vi "Measure all pixels on cell and save data.vi"(0 "Cell details cluster in":T1={"Measure?"=TRUE, "Area (cm^2)"=0.0, "Cell Label"="", "Cell Description"="", "Cell Position"=0, "Time in rig (s)"=0.0, "Time to next scan (s)"=0.0, "Scan number"=0.0, "When did you stick it in?"=0.0, "Time between scans (s)"=0.0, "Time of the last scan (s)"=0.0, "Scan settings in queue"=0, "Sample Holder"=0.0} {"Scan settings in queue" items=["Regular", "Inverted"]; "Time of the last scan (s)" format="%<%H:%M:%S>t"; "When did you stick it in?" format="%<%H:%M:%S>t"; "Time to next scan (s)" format="%<%H:%M:%S>t"; "Time in rig (s)" format="%<%H:%M:%S>t"}, 1 "Username":string, 5 "Cell Description":string, 6 "XYGraph Refnum":refnum<vi>, 7 "Cell position":dbl, 8 "Tbl Refnum":refnum<vi>, 9 "Sample Holder":dbl, 11 "Scan settings in queue":dbl, 12 "JV curve scan settings":T2(array[cluster])=[{"Light Intensity (Suns)"=1.0, "Stabilization Time (s)"=2.0, "Maximum Voltage (V)"=0.0, "Minimum Voltage (V)"=-1.4, "Range Options"=0, "Scan Direction\nDU (T), UD (F)"=FALSE, "Step Size (V)"=0.01, "Source Delay (s)"=0.001}, {"Light Intensity (Suns)"=1.0, "Stabilization Time (s)"=5.0, "Maximum Voltage (V)"=2.0, "Minimum Voltage (V)"=0.0, "Range Options"=0, "Scan Direction\nDU (T), UD (F)"=TRUE, "Step Size (V)"=0.04, "Source Delay (s)"=0.001}] {"Range Options" items=["Auto Range", "Semi-Auto Range", "100 uA", "1 mA", "10 mA", "100 mA", "1A"]}, 13 "Time Zero":timestamp) -> (4 "Cell details cluster out":T1={"Measure?"=TRUE, "Area (cm^2)"=0.0, "Cell Label"="", "Cell Description"="", "Cell Position"=0, "Time in rig (s)"=0.0, "Time to next scan (s)"=0.0, "Scan number"=0.0, "When did you stick it in?"=0.0, "Time between scans (s)"=0.0, "Time of the last scan (s)"=0.0, "Scan settings in queue"=0, "Sample Holder"=0.0} {"Scan settings in queue" items=["Regular", "Inverted"]; "Time of the last scan (s)" format="%<%H:%M:%S>t"; "When did you stick it in?" format="%<%H:%M:%S>t"; "Time to next scan (s)" format="%<%H:%M:%S>t"; "Time in rig (s)" format="%<%H:%M:%S>t"}, 15 "JV curve image path":path)   [LabVIEW 2011]
uses:
  <vilib>/ULx/Create Channel.llb/ULx Create Channel (DO-Digital Output).vi
  <vilib>/ULx/Write.llb/ULx Write (Digital U32 1Chan 1Samp).vi
  <instrlib>/keithley_24xx/Keithley 24XX/Keithley 24XX.lvlib
panel:
  in  "Tab Control 4":enum32{"Page 1"}(tab)
  out "JV Curve":cluster{"Y":dbl[], "Y":dbl[]}[](graph)
  in  "VISA resource name":refnum<visa-resource-name>="GPIB0::24::INSTR"
  in  "Port":refnum<k21>="Dev0/AuxPort"
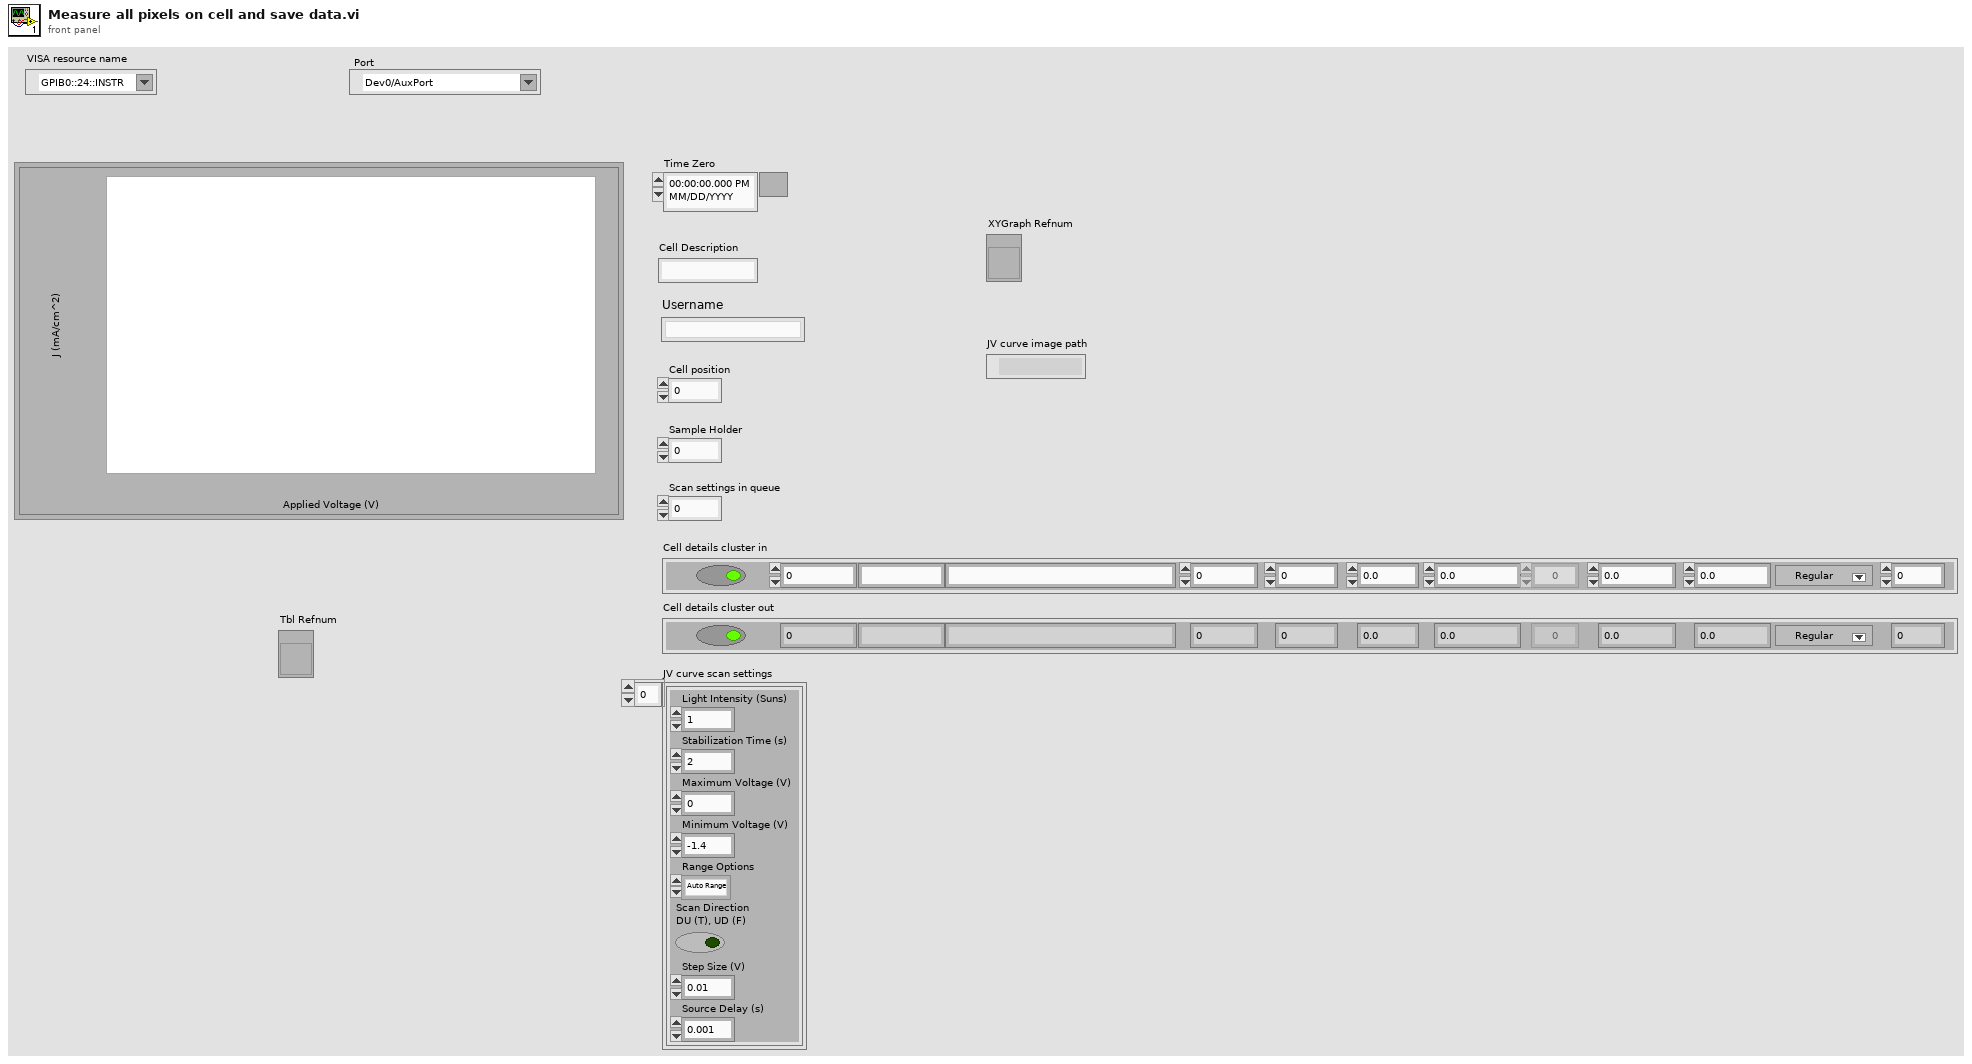
[diagram p1: front panel]
types:
  T1 = cluster{"Measure?":bool, "Area (cm^2)":dbl, "Cell Label":string, "Cell Description":string, "Cell Position":i32, "Time in rig (s)":dbl, "Time to next scan (s)":dbl, "Scan number":dbl, "When did you stick it in?":dbl, "Time between scans (s)":dbl, "Time of the last scan (s)":dbl, "Scan settings in queue":u16, "Sample Holder":dbl}
  T2 = cluster{"Light Intensity (Suns)":dbl, "Stabilization Time (s)":dbl, "Maximum Voltage (V)":dbl, "Minimum Voltage (V)":dbl, "Range Options":u16, "Scan Direction\nDU (T), UD (F)":bool, "Step Size (V)":dbl, "Source Delay (s)":dbl}[]
  T3 = cluster{"Light Intensity (Suns)":dbl, "Stabilization Time (s)":dbl, "Maximum Voltage (V)":dbl, "Minimum Voltage (V)":dbl, "Range Options":u16, "Scan Direction\nDU (T), UD (F)":bool, "Step Size (V)":dbl, "Source Delay (s)":dbl}
  T4 = typedef "imagedata.ctl" = cluster{"image type":i32, "image depth":i32, "image":u8[], "mask":u8[], "colors":u32[], "Rectangle":cluster{"left":i16, "top":i16, "right":i16, "bottom":i16}}
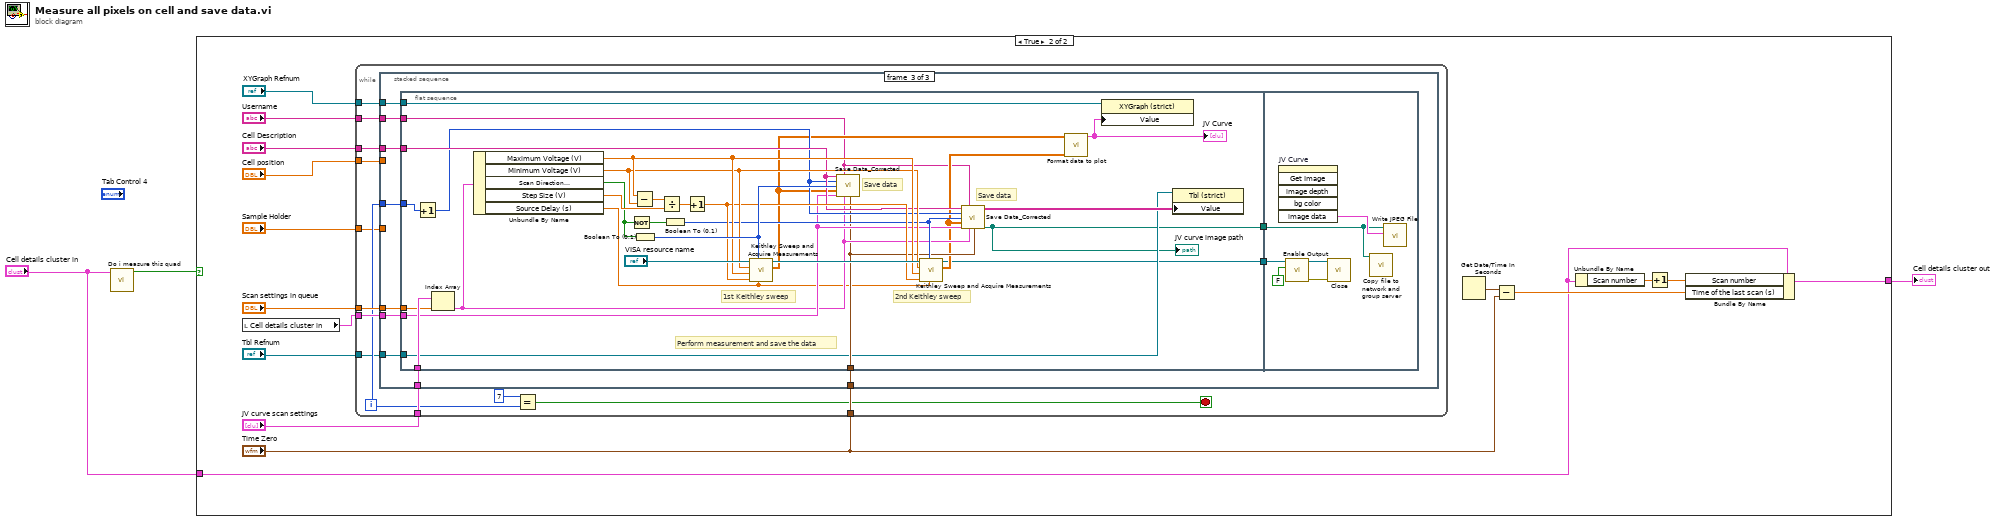
[diagram p0: block diagram]
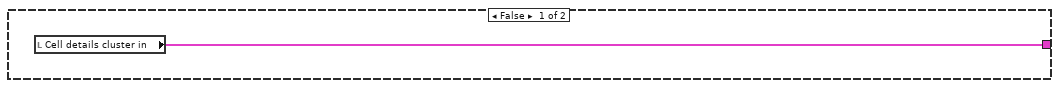
[diagram p2: hidden frame]
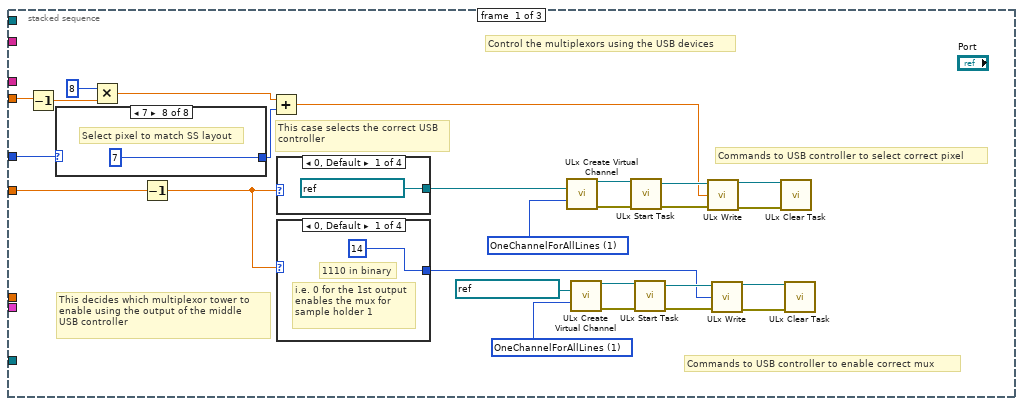
[diagram p3: hidden frame]
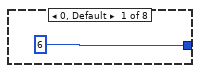
[diagram p4: hidden frame]
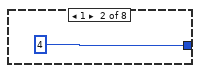
[diagram p5: hidden frame]
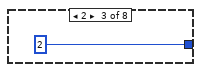
[diagram p6: hidden frame]
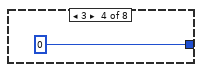
[diagram p7: hidden frame]
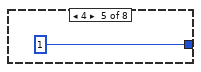
[diagram p8: hidden frame]
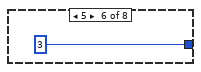
[diagram p9: hidden frame]
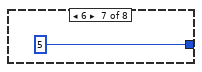
[diagram p10: hidden frame]
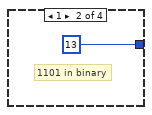
[diagram p11: hidden frame]
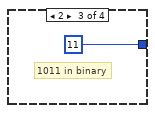
[diagram p12: hidden frame]
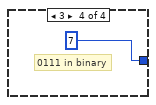
[diagram p13: hidden frame]
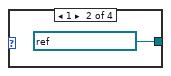
[diagram p14: hidden frame]
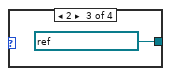
[diagram p15: hidden frame]
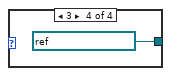
[diagram p16: hidden frame]
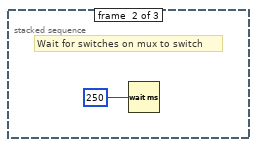
[diagram p17: hidden frame]
diagram:
  n1 = call "Do i measure this quad.vi"("Cell details"="Cell details cluster in") -> ("Measure cell?"=w3:bool)  [unwired: 10 in]
  n2 = case shown="True" w3 {
    tunnel: [w4 w9] -> w2
    tunnel: "Cell details cluster in" -> [_ w5]
    frame False {
      n3 = local read "Cell details cluster in"() -> (w4:T1)
    }
    frame True {
      n4 = local read "Cell details cluster in"() -> (w14:T1)
      n5 = while {
        tunnel: "JV curve scan settings" -> [w33]
        tunnel: "Scan settings in queue" -> [w32]
        tunnel: w14 -> [w31]
        tunnel: "Cell position" -> [w30]
        tunnel: "Sample Holder" -> [w27]
        tunnel: "Cell Description" -> [w26]
        tunnel: "Time Zero" -> [w25]
        tunnel: "Username" -> [w23]
        tunnel: "XYGraph Refnum" -> [w22]
        tunnel: "Tbl Refnum" -> [w21]
        i -> [w28]
        stop <- w24 stop-if-true
        n6 = stacked-sequence {
          tunnel: w33 -> [_ _ w87]
          tunnel: w32 -> [_ _ w86]
          tunnel: w31 -> [_ _ w83]
          tunnel: w30 -> [w49 _ _]
          tunnel: w28 -> [w35 _ w85]
          tunnel: w27 -> [w46 _ _]
          tunnel: w26 -> [_ _ w84]
          tunnel: w25 -> [_ _ w82]
          tunnel: w23 -> [_ _ w81]
          tunnel: w22 -> [_ _ w80]
          tunnel: w21 -> [_ _ w79]
          frame #0 {
            w45 = 1 items=["OneChannelForEachLine", "OneChannelForAllLines"] ("line grouping")
            w58 = 1 items=["OneChannelForEachLine", "OneChannelForAllLines"] ("line grouping")
            # "Control the multiplexors using the USB devices"
            # "Commands to USB controller to enable correct mux"
            # "Commands to USB controller to select correct pixel"
            # "This decides which multiplexor tower to\nenable using the output of the middle \nUSB controller"
            # "This case selects the correct USB\ncontroller"
            n7 = Decrement(x=w49) -> (x-1=w48:dbl)
            n8 = case shown="7" w35 {
              tunnel: [6 4 2 0 1 3 5 7] -> w34
              frame 0, Default {
              }
              frame 1 {
              }
              frame 2 {
              }
              frame 3 {
              }
              frame 4 {
              }
              frame 5 {
              }
              frame 6 {
              }
              frame 7 {
                # "Select pixel to match SS layout"
              }
            }
            n9 = Multiply(x=8, y=w48) -> (x*y=w50:dbl)
            n10 = Decrement(x=w46) -> (x-1=w37:dbl)
            n11 = Add(x=w50, y=w34) -> (x+y=w47:dbl)
            n12 = case shown="0, Default" w37 {
              tunnel: [refnum<k21> "Dev0/1stPortA" ("Port 2") refnum<k21> "Dev0/1stPortB" ("Port 2") refnum<k21> "Dev1/1stPortA" ("Port 2") refnum<k21> "Dev1/1stPortB" ("Port 2")] -> w59
              frame 0, Default {
              }
              frame 1 {
              }
              frame 2 {
              }
              frame 3 {
              }
            }
            n13 = case shown="0, Default" w37 {
              tunnel: [14 13 11 7] -> w36
              frame 0, Default {
                # "i.e. 0 for the 1st output\nenables the mux for\nsample holder 1"
                # "1110 in binary"
              }
              frame 1 {
                # "1101 in binary"
              }
              frame 2 {
                # "1011 in binary"
              }
              frame 3 {
                # "0111 in binary"
              }
            }
            n14 = call-poly <vilib>:"ULx Create Virtual Channel.vi"("lines"=w59, "line grouping"=w58) -> ("task out"=w56:refnum<k24>, "error out"=w57:errorcluster)  [unwired: 12 in]
            n15 = call-poly <vilib>:"ULx Create Virtual Channel.vi"("lines"=refnum<k21> "Dev2/1stPortA" ("Port 2"), "line grouping"=w45) -> ("task out"=w43:refnum<k24>, "error out"=w44:errorcluster)  [unwired: 12 in]
            n16 = call <vilib>:"ULx Start Task.vi"("task in"=w56, "error in"=w57) -> ("task out"=w53:refnum<k24>, "error out"=w52:errorcluster)  [unwired: 12 in]
            n17 = call <vilib>:"ULx Start Task.vi"("task in"=w43, "error in"=w44) -> ("task out"=w40:refnum<k24>, "error out"=w39:errorcluster)  [unwired: 12 in]
            n18 = call-poly <vilib>:"ULx Write.vi"("task in"=w53, "data"=w47, "error in"=w52) -> ("task out"=w55:refnum<k24>, "error out"=w54:errorcluster)  [unwired: 10 in, 1 out]
            n19 = call-poly <vilib>:"ULx Write.vi"("task in"=w40, "data"=w36, "error in"=w39) -> ("task out"=w42:refnum<k24>, "error out"=w41:errorcluster)  [unwired: 10 in, 1 out]
            n20 = call <vilib>:"ULx Clear Task.vi"("task in"=w55, "error in"=w54) -> ()  [unwired: 13 in, 1 out]
            n21 = call <vilib>:"ULx Clear Task.vi"("task in"=w42, "error in"=w41) -> ()  [unwired: 13 in, 1 out]
          }
          frame #1 {
            # "Wait for switches on mux to switch"
            n22 = Wait (ms)(milliseconds to wait=250) -> ()  [unwired: 1 out]
          }
          frame #2 {
            n23 = flat-sequence {
              tunnel: w87 -> [w116]
              tunnel: w86 -> [w115]
              tunnel: w85 -> [w108]
              tunnel: w84 -> [w103]
              tunnel: w83 -> [w100]
              tunnel: w82 -> [w98]
              tunnel: w81 -> [w94]
              tunnel: w80 -> [w93]
              tunnel: w79 -> [w91]
              tunnel: [w89] -> w78
              tunnel: [w88] -> w77
              tunnel: w78 -> [w122]
              tunnel: w77 -> [w118]
              frame #0 {
                # "Perform measurement and save the data"
                # "Save data"
                # "Save data"
                # "2nd Keithley sweep"
                # "1st Keithley sweep"
                n24 = Increment(x=w108) -> (x+1=w102:i32)
                n25 = Index Array(array=w116, index=w115) -> (element=w99:T3)
                n26 = Unbundle By Name(w99) -> ("Maximum Voltage (V)"=w106:dbl, "Minimum Voltage (V)"=w105:dbl, "Scan Direction\nDU (T), UD (F)"=w110:bool, "Step Size (V)"=w112:dbl, "Source Delay (s)"=w97:dbl)
                n27 = Not(x=w110) -> (.not. x?=w111:bool)
                n28 = Subtract(x=w106, y=w105) -> (x-y=w113:dbl)
                n29 = Boolean To (0,1)(Boolean=w110) -> (0, 1=w109:i16)
                n30 = Divide(x=w113, y=w112) -> (x/y=w114:dbl)
                n31 = Boolean To (0,1)(Boolean=w111) -> (0, 1=w101:i16)
                n32 = Increment(x=w114) -> (x+1=w104:dbl)
                n33 = call "Keithley Sweep and Acquire Measurements.vi"("Source Delay (s)"=w97, "Sweep Direction"=w109, "Number of Points"=w104, "Maximum Amplitude"=w106, "Minimum Amplitude"=w105, "VISA resource name"="VISA resource name") -> ("Data Array"=w96:dbl[][], "VISA resource name out"=w107:refnum<visa-resource-name>)  [unwired: 1 in, 1 out]
                n34 = call "Save Data_Corrected.vi"("Experiment Indicator"=w103, "Username"=w94, "Pixel"=w102, "Scan direction"=w109, "Data Array"=w96, "Cell details cluster"=w100, "Show me Scan \nSettings JV set"=w99, "Time zero"=w98) -> ()  [unwired: 3 in, 5 out]
                n35 = call "Keithley Sweep and Acquire Measurements.vi"("Source Delay (s)"=w97, "Sweep Direction"=w101, "Number of Points"=w104, "Maximum Amplitude"=w106, "Minimum Amplitude"=w105, "VISA resource name"=w107) -> ("Data Array"=w95:dbl[][], "VISA resource name out"=w88:refnum<visa-resource-name>)  [unwired: 1 in, 1 out]
                n36 = call "Save Data_Corrected.vi"("Experiment Indicator"=w103, "Username"=w94, "Pixel"=w102, "Scan direction"=w101, "Data Array"=w95, "Cell details cluster"=w100, "Show me Scan \nSettings JV set"=w99, "Time zero"=w98) -> ("Master Log"=w92:string[][], "File path for JV image"=w89:path)  [unwired: 3 in, 3 out]
                "JV curve image path" <- w89
                n37 = call "Format data to plot.vi"("Data Array 2"=w95, "Data Array"=w96) -> ("JV Curve"=w90:cluster{"Y":dbl[], "Y":dbl[]}[])  [unwired: 9 in]
                "JV Curve" <- w90
                n38 = property class="XYGraph (strict)"(reference=w93, "Value"=w90) -> ()  [unwired: 1 in, 2 out]
                n39 = property class="Tbl (strict)"(reference=w91, "Value"=w92) -> ()  [unwired: 1 in, 2 out]
              }
              frame #1 {
                n40 = invoke on="JV Curve" class="XYGraph (strict)" method="Get Image"() -> ("image data"=w123:T4)  [unwired: 6 in, 5 out]
                n41 = call <instrlib>:"Enable Output.vi"("Enable Output (T: Enable)"=FALSE, "VISA resource name"=w118) -> ("error out"=w120:errorcluster, "VISA resource name out"=w119:refnum<visa-resource-name>)  [unwired: 8 in]
                n42 = call <instrlib>:"Close.vi"("error in (no error)"=w120, "VISA resource name"=w119) -> ()  [unwired: 9 in, 1 out]
                n43 = call "Copy file to network and group server.vi"("File path in"=w122) -> ()  [unwired: 11 in]
                n44 = call <vilib>:"Write JPEG File.vi"("image data"=w123, "path to JPEG file"=w122) -> ()  [unwired: 8 in, 2 out]
              }
            }
          }
        }
        n45 = Equal?(x=7, y=w28) -> (x = y?=w24:bool)
      }
      n46 = Get Date/Time In Seconds() -> (seconds since 1Jan1904=w13:timestamp)
      n47 = Subtract(x=w13, y="Time Zero") -> (x-y=w8:dbl)
      n48 = Unbundle By Name(w5) -> ("Scan number"=w10:dbl)
      n49 = Increment(x=w10) -> (x+1=w11:dbl)
      n50 = Bundle By Name(cluster=w5, "Scan number"=w11, "Time of the last scan (s)"=w8) -> (w9:T1)
    }
  }
  "Cell details cluster out" <- w2
